vi "Filter Vision Model.vi"(11 "Available Models":string[](array[string])) -> (3 "Model Rings":cluster{"String":string, "Value":string}[](array[cluster]))   [LabVIEW 2023, in "LabVIEW LLM.lvlib"]
uses:
  LabVIEW LLM.lvlib
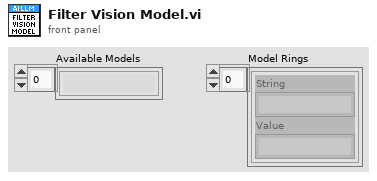
[diagram p1: front panel]
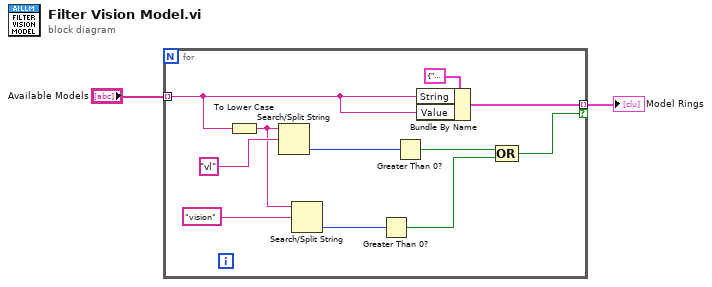
[diagram p0: block diagram]
diagram:
  n1 = for {
    tunnel: [w12] -> w1 mode=indexing if=w4
    tunnel: "Available Models" -> [w11] mode=indexing
    n2 = To Lower Case(string=w11) -> (all lower case string=w6:string)
    n3 = Search/Split String(string=w6, search string/char (-)="vl") -> (offset of match=w9:i32)  [unwired: 1 in, 2 out]
    n4 = Search/Split String(string=w6, search string/char (-)="vision") -> (offset of match=w5:i32)  [unwired: 1 in, 2 out]
    n5 = Greater Than 0?(x=w5) -> (x > 0?=w3:bool)
    n6 = Greater Than 0?(x=w9) -> (x > 0?=w8:bool)
    n7 = Bundle By Name(cluster=cluster{"String":string, "Value":string} {"String"="", "Value"=""} ("Cluster"), "String"=w11, "Value"=w11) -> (w12:cluster{"String":string, "Value":string})
    n8 = Compound Arithmetic op=OR(w8, w3) -> (w4:bool)
  }
  "Model Rings" <- w1
